vi "set_dds.vi"(6 "DDS board initialization parameters":T2={"Bypass PLL"=FALSE, "PLL Range"=TRUE, "Update Clock"=FALSE, "Triangle "=FALSE, "SDO Active"=FALSE, "LSB First"=FALSE, "OSK Int"=FALSE, "Output Shaped Keying Enable"=TRUE, "Bypass Sinc"=FALSE, "Digital Part"=TRUE, "OutPut DAC"=TRUE, "Control DAC"=TRUE, "Comparator"=FALSE, "Modus"=0, "Multiplier Value"=15} {"Modus" scale=0.0..4.0}, 7 "update?":bool, 8 "error in (no error)":errorcluster, 9 "inverse?":T1(ring), 10 "OSK select":bool=TRUE, 11 "FPGAWrapperMH120124FrameScan_PXI7813R in":refnum<class "FPGAWrapperMH120124FrameScan_PXI7813R.lvclass">) -> (0 "error out":errorcluster, 3 "FPGAWrapperMH120124FrameScan_PXI7813R out":refnum<class "FPGAWrapperMH120124FrameScan_PXI7813R.lvclass">)   [LabVIEW 2010, in "FPGAWrapperMH120124FrameScan_PXI7813R.lvclass"]
uses:
  FPGAWrapperMH120124FrameScan_PXI7813R.lvclass
  fpgaVIsAndControls/DDS_board_init_cluster.ctl
  FPGAWrapperMH120124FrameScan_PXI7813R.lvclass/FPGAWrapperMH120124FrameScan_PXI7813R.ctl
panel:
  # "FSK"
  # "Ramped"
  # "FSK"
  # "Chirp Modus"
  # "Unramped"
  # "BPSK"
  # "Single Tone"
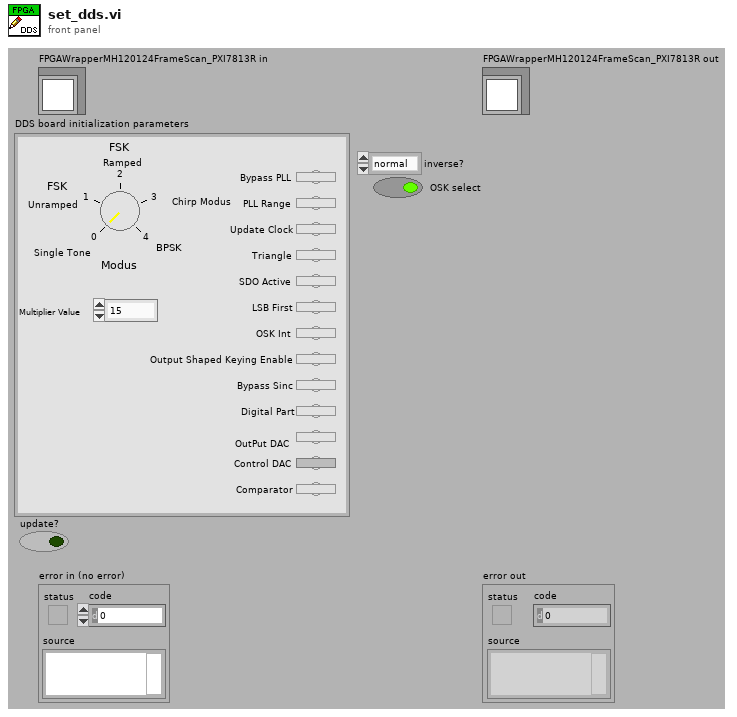
[diagram p1: front panel]
types:
  T1 = enum16{"normal", "x inversed", "y inversed", "x & y inversed"}
  T2 = typedef "DDS_board_init_cluster.ctl" = cluster{"Bypass PLL":bool, "PLL Range":bool, "Update Clock":bool, "Triangle ":bool, "SDO Active":bool, "LSB First":bool, "OSK Int":bool, "Output Shaped Keying Enable":bool, "Bypass Sinc":bool, "Digital Part":bool, "OutPut DAC":bool, "Control DAC":bool, "Comparator":bool, "Modus":u8, "Multiplier Value":u8}
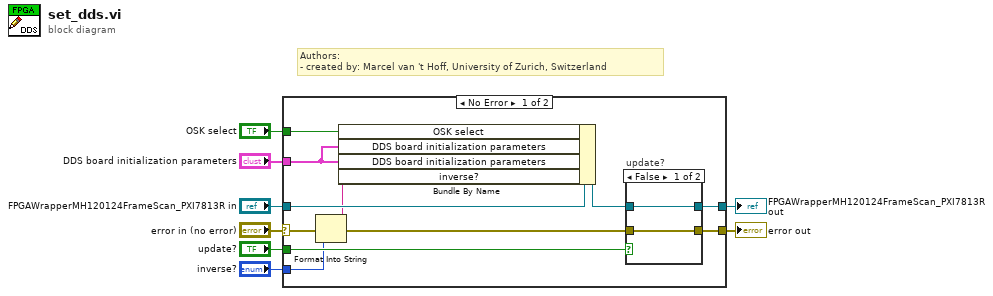
[diagram p0: block diagram]
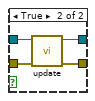
[diagram p2: hidden frame]
diagram:
  # "Authors: \n- created by: Marcel van 't Hoff, University of Zurich, Switzerland"
  n1 = case shown="No Error" "error in (no error)" {
    selector: "error in (no error)" -> [w11 w27]
    tunnel: [w16 w27] -> w7
    tunnel: [w17 w26] -> w5
    tunnel: "FPGAWrapperMH120124FrameScan_PXI7813R in" -> [w19 w26]
    tunnel: "DDS board initialization parameters" -> [w15 _]
    tunnel: "inverse?" -> [w12 _]
    tunnel: "OSK select" -> [w14 _]
    tunnel: "update?" -> [w13 _]
    frame No Error {
      n2 = Format Into String(error in=w11, w12) -> (resulting string=w9:string, error out=w10:errorcluster)  [unwired: 2 in]
      n3 = Bundle By Name(cluster=w19, "OSK select"=w14, "DDS board initialization parameters"=w15, "DDS board initialization parameters"=w15, "inverse?"=w9) -> (w18:refnum<class "FPGAWrapperMH120124FrameScan_PXI7813R.lvclass">)
      n4 = case "update?" shown="False" w13 {
        tunnel: w18 -> [w20 w25]
        tunnel: [w20 w24] -> w17
        tunnel: w10 -> [w21 w23]
        tunnel: [w21 w22] -> w16
        frame False {
        }
        frame True {
          n5 = call-dynamic "update.vi"("error in (no error)"=w23, "FPGAWrapperMH120124FrameScan_PXI7813R in"=w25) -> ("error out"=w22:errorcluster, "FPGAWrapperMH120124FrameScan_PXI7813R out"=w24:refnum<class "FPGAWrapperMH120124FrameScan_PXI7813R.lvclass">)  [unwired: 8 in]
        }
      }
    }
    frame Error {
    }
  }
  "error out" <- w7
  "FPGAWrapperMH120124FrameScan_PXI7813R out" <- w5
